vi "Threshold 1D Array (Linear Search) [DBL].vi"(0 "Array":dbl[](array[numeric]), 2 "Y":dbl, 3 "start index (0)":i32) -> (7 "fractional index":dbl)   [LabVIEW 2021, in "Arrays.lvlib"]
uses:
  Arrays.lvlib
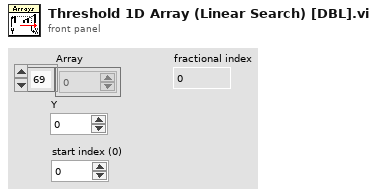
[diagram p1: front panel]
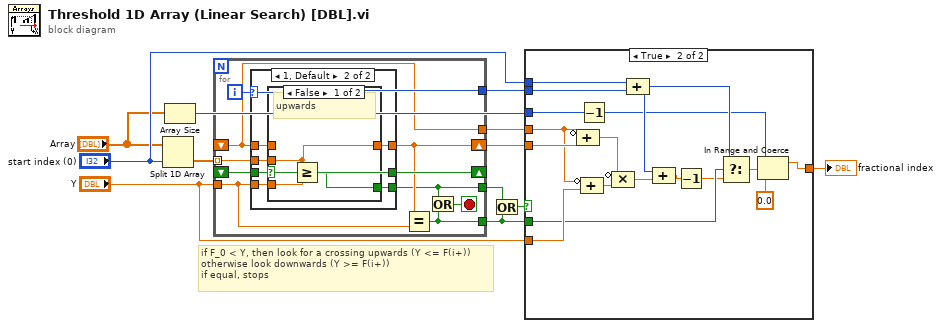
[diagram p0: block diagram]
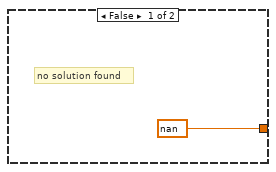
[diagram p2: hidden frame]
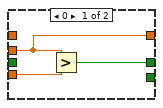
[diagram p3: hidden frame]
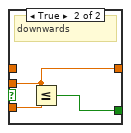
[diagram p4: hidden frame]
diagram:
  # "if F_0 < Y, then look for a crossing upwards (Y <= F(i+))\notherwise look downwards (Y >= F(i+))\nif equal, stops"
  n1 = Split 1D Array(array="Array", index="start index (0)") -> (second subarray=w12:dbl[])  [unwired: 1 out]
  n2 = Array Size(array="Array") -> (size(s)=w1:i32)
  n3 = for {
    tunnel: w12 -> [w21] mode=indexing
    tunnel: "Y" -> [w18]
    shift-right: [w22] -> _
    shift-left: _ -> [w20]
    shift-right: [w19] -> w10
    shift-left: _ -> [w13]
    tunnel: [w17] -> w9
    tunnel: [w15] -> w7
    tunnel: [w14] -> w5
    tunnel: [w13] -> w4
    i -> [w17]
    stop <- w16 stop-if-true
    n4 = case shown="1, Default" w17 {
      tunnel: w21 -> [w24 w31]
      tunnel: w18 -> [w23 w30]
      tunnel: [w25 w29] -> w22
      tunnel: w20 -> [_ w29]
      tunnel: [w24 w27] -> w19
      tunnel: [_ w28] -> w15
      tunnel: w13 -> [_ w26]
      frame 0 {
        n5 = Greater?(x=w24, y=w23) -> (0:w25:bool)
      }
      frame 1, Default {
        n6 = case shown="False" w29 {
          tunnel: w31 -> [w32 w35]
          tunnel: w30 -> [w34 w37]
          tunnel: [w33 w36] -> w28
          tunnel: [w32 w35] -> w27
          tunnel: w26 -> [_ _]
          frame False {
            # "upwards"
            n7 = Greater Or Equal?(x=w32, y=w34) -> (x >= y?=w33:bool)
          }
          frame True {
            # "downwards"
            n8 = Less Or Equal?(x=w35, y=w37) -> (x <= y?=w36:bool)
          }
        }
      }
    }
    n9 = Equal?(x=w19, y=w18) -> (x = y?=w14:bool)
    n10 = Or(x=w15, y=w14) -> (x .or. y?=w16:bool)
  }
  n11 = Or(x=w7, y=w5) -> (x .or. y?=w6:bool)
  n12 = case shown="True" w6 {
    tunnel: "Y" -> [_ w55]
    tunnel: w10 -> [_ w46]
    tunnel: w9 -> [_ w49]
    tunnel: [nan w42] -> w8
    tunnel: w5 -> [_ w50]
    tunnel: w4 -> [_ w45]
    tunnel: "start index (0)" -> [_ w43]
    tunnel: w1 -> [_ w41]
    frame False {
      # "no solution found"
    }
    frame True {
      n13 = Compound Arithmetic op=ADD(invert w45, w46) -> (w54:dbl)
      n14 = Decrement(x=w41) -> (x-1=w39:i32)
      n15 = Compound Arithmetic op=ADD(invert w45, w55) -> (w53:dbl)
      n16 = Compound Arithmetic op=MULTIPLY(invert w54, w53) -> (w52:dbl)
      n17 = Compound Arithmetic op=ADD(w43, w49) -> (w44:i32)
      n18 = Compound Arithmetic op=ADD(w44, w52) -> (w51:dbl)
      n19 = Decrement(x=w51) -> (x-1=w48:dbl)
      n20 = Select(t=w44, s=w50, f=w48) -> (s? t:f=w47:dbl)
      n21 = In Range and Coerce(upper limit=w39, x=w47, lower limit=0.0) -> (coerced(x)=w42:dbl)  [unwired: 1 out]
    }
  }
  "fractional index" <- w8
